vi "HTS_PLATEMAP_TO_WELL_LIST.vi"(10 "PLATE_MAP":T4=[[FALSE, FALSE, FALSE, FALSE, FALSE, FALSE, FALSE, TRUE, FALSE, FALSE, FALSE, FALSE], [FALSE, FALSE, FALSE, FALSE, FALSE, FALSE, FALSE, FALSE, FALSE, FALSE, FALSE, FALSE], [FALSE, FALSE, FALSE, FALSE, FALSE, FALSE, FALSE, FALSE, FALSE, FALSE, FALSE, FALSE], [FALSE, FALSE, FALSE, FALSE, FALSE, FALSE, FALSE, FALSE, FALSE, FALSE, FALSE, FALSE], [FALSE, FALSE, FALSE, FALSE, FALSE, FALSE, FALSE, FALSE, FALSE, FALSE, FALSE, FALSE], [FALSE, FALSE, FALSE, FALSE, FALSE, FALSE, FALSE, FALSE, FALSE, FALSE, FALSE, FALSE], [FALSE, FALSE, FALSE, FALSE, FALSE, FALSE, FALSE, FALSE, FALSE, FALSE, FALSE, FALSE], [FALSE, FALSE, FALSE, FALSE, FALSE, FALSE, FALSE, FALSE, FALSE, FALSE, FALSE, FALSE]]) -> (2 "WELL_LIST":T1[](array[typedef]))   [LabVIEW 2009]
uses:
  HTS_PLATE_DISPLAY.ctl
  HTS_WELL.ctl
  HTS_COLUMN.ctl
  HTS_ROW.ctl
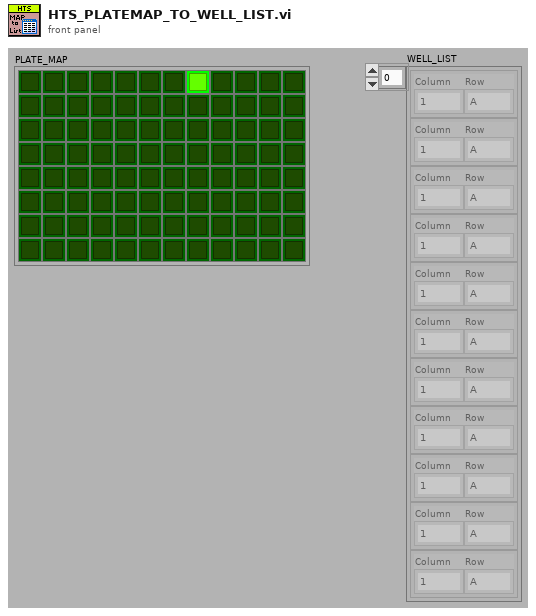
[diagram p1: front panel]
types:
  T1 = typedef "HTS_WELL.ctl" = cluster{"Column":T2, "Row":T3}
  T2 = typedef "HTS_COLUMN.ctl" = enum16{"1", "2", "3", "4", "5", "6", "7", "8", "9", "10", "11", "12"}
  T3 = typedef "HTS_ROW.ctl" = enum16{"A", "B", "C", "D", "E", "F", "G", "H"}
  T4 = typedef "HTS_PLATE_DISPLAY.ctl" = bool[][]
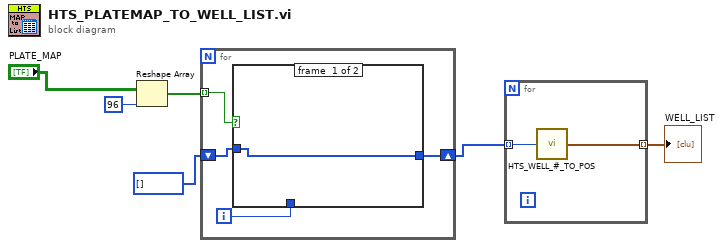
[diagram p0: block diagram]
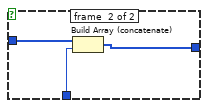
[diagram p2: hidden frame]
diagram:
  n1 = Reshape Array("PLATE_MAP", 96 ("dimension size")) -> (w4:bool[])
  n2 = for {
    tunnel: w4 -> [w10] mode=indexing
    shift-right: [w8] -> w2
    shift-left: i32[] [] -> [w7]
    i -> [w9]
    n3 = case shown="True" w10 {
      tunnel: w9 -> [_ w14]
      tunnel: [w11 w13] -> w8
      tunnel: w7 -> [w11 w12]
      frame #0 {
      }
      frame #1 {
        n4 = Build Array (concatenate)(w12, w14) -> (w13:i32[])
      }
    }
  }
  n5 = for {
    tunnel: w2 -> [w16] mode=indexing
    tunnel: [w15] -> w1 mode=indexing
    n6 = call "HTS_WELL_#_TO_POS.vi"("Well Number (0-95)"=w16) -> ("Well Position"=w15:T1)  [unwired: 4 in]
  }
  "WELL_LIST" <- w1
